vi "User@TextRingBlinking__Parameter.vi"(1 "ParamterIn":string) -> (0 "ParamterOut":string)   [LabVIEW 2019]
panel:
  in  "Parameters":string(combo)
  in  "UserPanelControl":string(combo)
  in  "Confirm":bool
  # "User@TextRingBlinking $UserPanelControlName,$Logic"
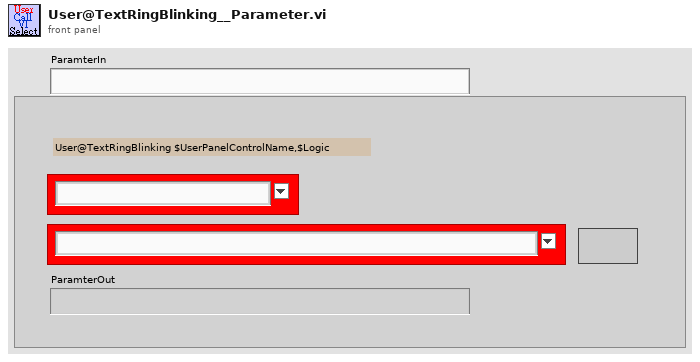
[diagram p1: front panel]
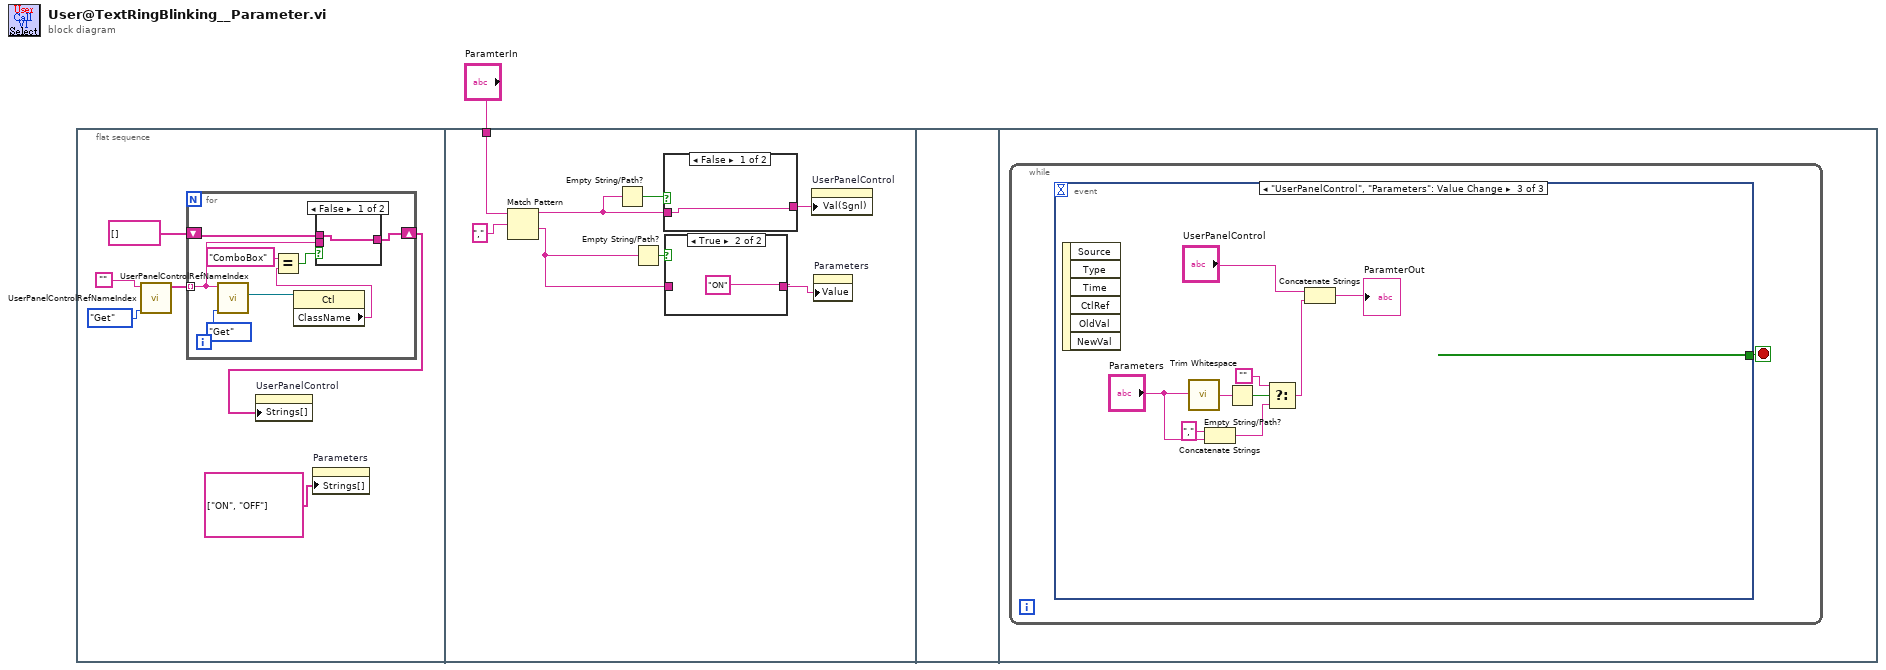
[diagram p0: block diagram]
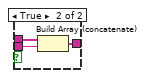
[diagram p2: hidden frame]
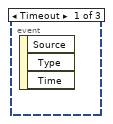
[diagram p5: hidden frame]
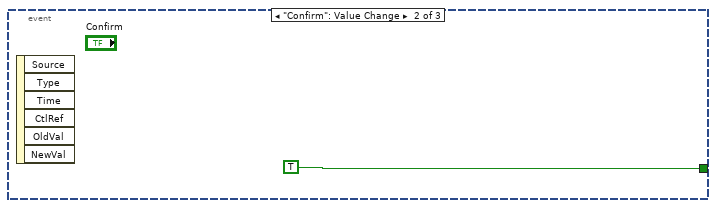
[diagram p6: hidden frame]
diagram:
  n1 = flat-sequence {
    tunnel: "ParamterIn" -> [w25]
    frame #0 {
      n2 = call "UserPanelControlRefNameIndex.vi"("OP"=enum16{"Get", "Update", "Init"}."Get", "ControlName"="") -> ("ControlNameS"=w5:string[])  [unwired: 6 in, 3 out]
      n3 = for {
        tunnel: w5 -> [w10] mode=indexing
        shift-right: [w9] -> w3
        shift-left: string[] [] ("Strings []") -> [w11]
        n4 = call "UserPanelControlRefNameIndex.vi"("OP"=enum16{"Get", "Update", "Init"}."Get", "ControlName"=w10) -> ("ControlRefOut"=w14:refnum<vi>)  [unwired: 6 in, 3 out]
        n5 = property class="Ctl"(reference=w14) -> ("ClassName"=w13:string)  [unwired: 1 in, 2 out]
        n6 = Equal?(x="ComboBox" ("Class Name"), y=w13) -> (x = y?=w12:bool)
        n7 = case shown="False" w12 {
          tunnel: w11 -> [w16 w19]
          tunnel: w10 -> [_ w18]
          tunnel: [w16 w17] -> w9
          frame False {
          }
          frame True {
            n8 = Build Array (concatenate)(w19, w18) -> (w17:string[])
          }
        }
      }
      n9 = property on="UserPanelControl" class="CmbBox"("Strings[]"=w3) -> ()  [unwired: 2 in, 2 out]
      n10 = property on="Parameters" class="CmbBox"("Strings[]"=string[] ["ON", "OFF"] ("Strings []")) -> ()  [unwired: 2 in, 2 out]
    }
    frame #1 {
      n11 = Match Pattern(string=w25, regular expression=",") -> (before substring=w23:string, after substring=w22:string)  [unwired: 1 in, 2 out]
      n12 = Empty String/Path?(string/path=w23) -> (empty?=w27:bool)
      n13 = Empty String/Path?(string/path=w22) -> (empty?=w26:bool)
      n14 = case shown="False" w27 {
        tunnel: w23 -> [w30 w31]
        tunnel: [w30 w31] -> w20
        frame False {
        }
        frame True {
        }
      }
      n15 = case shown="True" w26 {
        tunnel: [w28 "ON"] -> w21
        tunnel: w22 -> [w28 _]
        frame False {
        }
        frame True {
        }
      }
      n16 = property on="UserPanelControl" class="CmbBox"("Val(Sgnl)"=w20) -> ()  [unwired: 2 in, 2 out]
      n17 = property on="Parameters" class="CmbBox"("Value"=w21) -> ()  [unwired: 2 in, 2 out]
    }
    frame #2 {
    }
    frame #3 {
      n18 = while {
        stop <- w32 stop-if-true
        n19 = event shown="[2] \"UserPanelControl\", \"Parameters\": Value Change" {
          selector: _ -> [_ _ _]
          dyn-events: _ -> [_ _ _]
          timeout: _ -> [_ _ _]
          tunnel: [_ TRUE _] -> w32
          event Timeout {
            n20 = event-data() -> ()  [unwired: 1 in, 3 out]
          }
          event "Confirm": Value Change {
            n21 = event-data() -> ()  [unwired: 1 in, 6 out]
          }
          event "UserPanelControl", "Parameters": Value Change {
            n22 = event-data() -> ()  [unwired: 1 in, 6 out]
            n23 = call <vilib>:"Trim Whitespace.vi"("string"="Parameters") -> ("trimmed string"=w38:string)  [unwired: 1 in]
            n24 = Concatenate Strings("," ("string"), "Parameters") -> (w37:string)
            n25 = Empty String/Path?(string/path=w38) -> (empty?=w39:bool)
            n26 = Select(t="", s=w39, f=w37) -> (s? t:f=w34:string)
            n27 = Concatenate Strings("UserPanelControl", w34) -> (→"ParamterOut":string)
          }
        }
      }
    }
  }
